vi "Resource Location.vi"() -> (2 "Resource Location":path)   [LabVIEW 2020, in "RxnRover.lvlib" / "File IO.lvlib" / "Project Locations.lvlib"]
doc: "Returns the resource location for the application, independent of whether it is run with the LabVIEW runtime, as a standalone EXE, using an installer, or during development in LabVIEW."
uses:
  Project Locations.lvlib
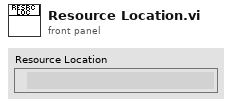
[diagram p1: front panel]
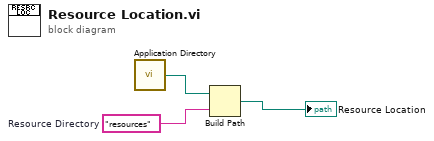
[diagram p0: block diagram]
diagram:
  w2 = "resources"  # Resource Directory
  n1 = call <vilib>:"Application Directory.vi"() -> ("Application Directory"=w3:path)
  n2 = Build Path(base path=w3, name or relative path=w2) -> (appended path=→"Resource Location":path)
